vi "Script_InlineAll.vi"() -> ()   [LabVIEW 2024]
panel:
  out "Current File":path
  out "error out":errorcluster
  out "All Files":path[](array[path])
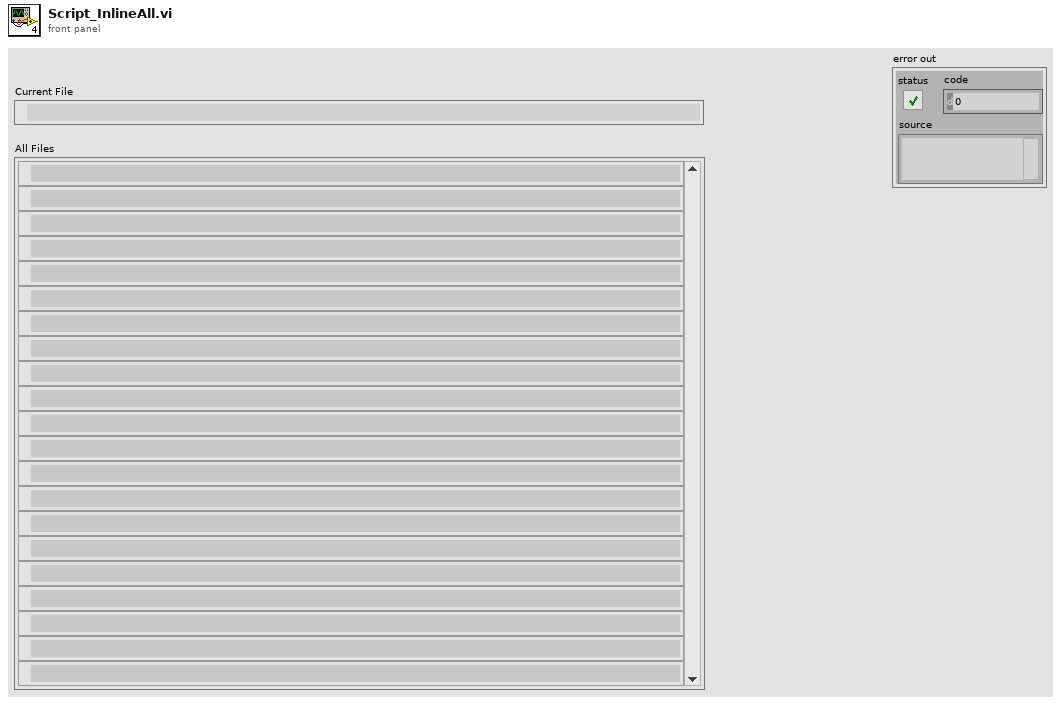
[diagram p1: front panel]
types:
  T1 = enum16{"Share clones between instances", "Preallocate clone for each instance"}
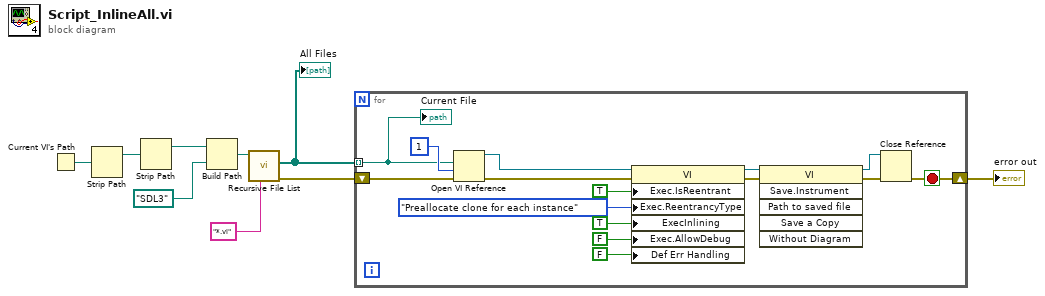
[diagram p0: block diagram]
diagram:
  n1 = Current VI's Path() -> (path=w9:path)
  n2 = Strip Path(path=w9) -> (stripped path=w8:path)  [unwired: 1 out]
  n3 = Strip Path(path=w8) -> (stripped path=w4:path)  [unwired: 1 out]
  n4 = Build Path(base path=w4, name or relative path=path "SDL3") -> (appended path=w6:path)
  n5 = call <vilib>:"Recursive File List.vi"("pattern"="*.vi", "Folder Path"=w6) -> ("error out"=w2:errorcluster, "All Files in Dir"=w3:path[])  [unwired: 5 in, 3 out]
  "All Files" <- w3
  n6 = for {
    tunnel: w3 -> [w10] mode=indexing
    shift-right: [w13] -> w1
    shift-left: w2 -> [w23]
    stop <- w13 stop-if-true
    n7 = Open VI Reference(vi path=w10, options=1, error in (no error)=w23) -> (vi reference=w20:refnum<vi>, error out=w22:errorcluster)  [unwired: 3 in]
    n8 = property class="VI"(reference=w20, error in=w22, "Exec.IsReentrant"=TRUE ("Execution:Is Reentrant"), "Exec.ReentrancyType"=T1."Preallocate clone for each instance" ("Execution:Reentrancy Type"), "ExecInlining"=TRUE ("Execution:Inline SubVI"), "Exec.AllowDebug"=FALSE ("Execution:Allow Debugging"), "Def Err Handling"=FALSE ("Automatic Error Handling")) -> (reference out=w15:refnum<vi>, error out=w21:errorcluster)
    n9 = invoke class="VI" method="Save.Instrument"(reference=w15, error in=w21) -> (reference out=w14:refnum<vi>, error out=w16:errorcluster)  [unwired: 4 in, 4 out]
    n10 = Close Reference(reference=w14, error in (no error)=w16) -> (error out=w13:errorcluster)
    "Current File" <- w10
  }
  "error out" <- w1
